vi "Remove Duplicates from Offsprings.vi"(11 "OffSpring":T1[](array[typedef])) -> (3 "Offspring with No Duplicates":T1[](array[typedef]))   [LabVIEW 2013, in "GA.lvclass"]
uses:
  GA.lvclass
  Controls/Solution_GA.ctl
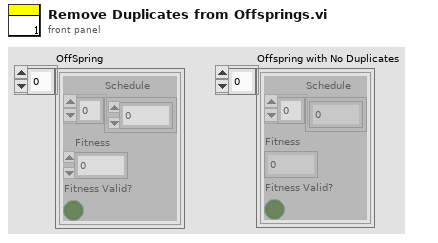
[diagram p1: front panel]
types:
  T1 = typedef "Solution_GA.ctl" = cluster{"Schedule":u16[], "Fitness":u16, "Fitness Valid?":bool}
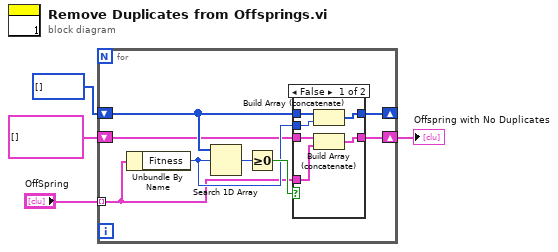
[diagram p0: block diagram]
diagram:
  n1 = for {
    tunnel: "OffSpring" -> [w6] mode=indexing
    shift-right: [w8] -> _
    shift-left: u16[] [] -> [w10]
    shift-right: [w5] -> w4
    shift-left: T1[] [] -> [w7]
    n2 = Unbundle By Name(w6) -> ("Fitness"=w9:u16)
    n3 = Search 1D Array(1D array=w10, element=w9) -> (index of element=w12:i32)  [unwired: 1 in]
    n4 = Greater Or Equal To 0?(x=w12) -> (x >= 0?=w11:bool)
    n5 = case shown="False" w11 {
      tunnel: w10 -> [w18 w20]
      tunnel: w9 -> [w17 _]
      tunnel: [w16 w20] -> w8
      tunnel: w7 -> [w15 w19]
      tunnel: w6 -> [w14 _]
      tunnel: [w13 w19] -> w5
      frame False {
        n6 = Build Array (concatenate)(w18, w17) -> (w16:u16[])
        n7 = Build Array (concatenate)(w15, w14) -> (w13:T1[])
      }
      frame True {
      }
    }
  }
  "Offspring with No Duplicates" <- w4
